vi "Get_Statistic.vi"(4 "Plot Data":T1) -> (1 "Chosen Statistic":dbl[](array[numeric]))   [LabVIEW 2022 SP3]
uses:
  Controls/Stats_Menu.ctl
  Globals/Meas_global.vi
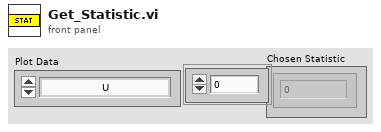
[diagram p1: front panel]
types:
  T1 = typedef "Stats_Menu.ctl" = enum16{"U", "u^2", "u^3", "u^4", "Skew_u", "Kurt_u", "% u'/U"}
  T2 = typedef "Analysis_info_cluster.ctl" = cluster{"Colour":u32, "Inst type":T3, "Inst name":string, "Symbol":string, "Code name":string, "Extra Info":string, "Inst Array":T4, "Extra Titles":string[], "Extra Values":string[], "U":dbl, "u^2":dbl, "u^3":dbl, "u^4":dbl, "Skew_u":dbl, "Kurt_u":dbl, "Sd Error in Mean":dbl, "% u'/U":dbl, "X":dbl, "Y":dbl, "Z":dbl, "Timescale integral Estimate":dbl, "Sd Error in Variance":dbl, "Calib File":path, "Calib Constants":dbl[], "Output Position":bool, "Stats":enum16{"None", "Basic", "Full"}, "Av Sampling Rate":dbl, "Av No of Samples":dbl, "Total Meas Time (s)":dbl, "ADAM Ch Name":string, "Max value":dbl, "Min value":dbl, "Req Sample Rate Hz":dbl, "Sync Delay Time (s)":dbl, "Ch No":i16, "Device":string, "Use Latest Calib":bool, "Port":string, "Metadata Ch Names":string[], "Metadata Ch Values":string[], "Label":string}
  T3 = typedef "Inst_type.ctl" = enum16{"Raw voltage", "Raw with zero offsetting", "Propeller anemometer", "Pressure Transducer", "Pitot-static tube", "Hot wire", "Cross wire 1", "Cross wire 2", "Generic Linear", "Generic Polynomial", "Generic BackPoly", "Fast FID", "Thermocouple", "Cold wire", "Pulsed Wire", "LDA Vel", "LDA Tran time", "LDA Arr time", "Microphone"}
  T4 = typedef "Instrument_Array.ctl" = enum16{"PWA", "LDA", "Analogue"}
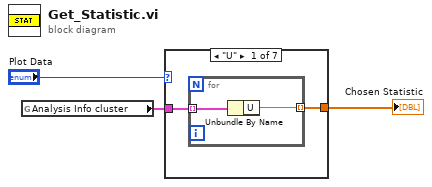
[diagram p0: block diagram]
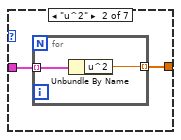
[diagram p2: hidden frame]
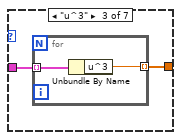
[diagram p3: hidden frame]
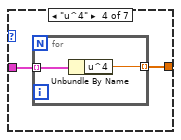
[diagram p4: hidden frame]
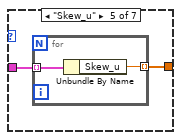
[diagram p5: hidden frame]
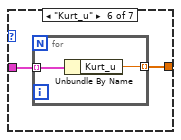
[diagram p6: hidden frame]
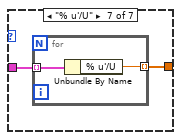
[diagram p7: hidden frame]
diagram:
  n1 = global read "Meas_global.vi" "Analysis Info cluster"() -> (w2:T2[])
  n2 = case shown="\"U\"" "Plot Data" {
    tunnel: w2 -> [w5 w9 w13 w17 w21 w25 w29]
    tunnel: [w4 w8 w12 w16 w20 w24 w28] -> w1
    frame "U" {
      n3 = for {
        tunnel: w5 -> [w7] mode=indexing
        tunnel: [w6] -> w4 mode=indexing
        n4 = Unbundle By Name(w7) -> ("U"=w6:dbl)
      }
    }
    frame "u^2" {
      n5 = for {
        tunnel: w9 -> [w11] mode=indexing
        tunnel: [w10] -> w8 mode=indexing
        n6 = Unbundle By Name(w11) -> ("u^2"=w10:dbl)
      }
    }
    frame "u^3" {
      n7 = for {
        tunnel: w13 -> [w15] mode=indexing
        tunnel: [w14] -> w12 mode=indexing
        n8 = Unbundle By Name(w15) -> ("u^3"=w14:dbl)
      }
    }
    frame "u^4" {
      n9 = for {
        tunnel: w17 -> [w19] mode=indexing
        tunnel: [w18] -> w16 mode=indexing
        n10 = Unbundle By Name(w19) -> ("u^4"=w18:dbl)
      }
    }
    frame "Skew_u" {
      n11 = for {
        tunnel: w21 -> [w23] mode=indexing
        tunnel: [w22] -> w20 mode=indexing
        n12 = Unbundle By Name(w23) -> ("Skew_u"=w22:dbl)
      }
    }
    frame "Kurt_u" {
      n13 = for {
        tunnel: w25 -> [w27] mode=indexing
        tunnel: [w26] -> w24 mode=indexing
        n14 = Unbundle By Name(w27) -> ("Kurt_u"=w26:dbl)
      }
    }
    frame "% u'/U" {
      n15 = for {
        tunnel: w29 -> [w31] mode=indexing
        tunnel: [w30] -> w28 mode=indexing
        n16 = Unbundle By Name(w31) -> ("% u'/U"=w30:dbl)
      }
    }
  }
  "Chosen Statistic" <- w1
